vi "Test in Loop.vi"() -> ()   [LabVIEW 2025]
uses:
  99_Reference/LVMQTT-master/Controls/Connection_Return_Codes.ctl
  99_Reference/LVMQTT-master/Controls/User_Info.ctl
  99_Reference/LVMQTT-master/Controls/Connect_Flags.ctl
  99_Reference/LVMQTT-master/Controls/QoS.ctl
  99_Reference/LVMQTT-master/Controls/DUP_Flag.ctl
  99_Reference/LVMQTT-master/Controls/Retain_Flag.ctl
  <vilib>/NI/AMC/Read Termination Message.vi
  <vilib>/NI/AMC/Create Single Message.vi
  <vilib>/NI/AMC/Update Message Routing Info.vi
  <vilib>/NI/AMC/Globals.vi
  <vilib>/NI/AMC/Send Message.vi
  <vilib>/ErrorRing/Error Ring.xnode
  99_Reference/LVMQTT-master/MQTT_Functions.lvlib
  <vilib>/NI/AMC/AMC.lvlib
  <userlib>/_OpenG.lib/time/time.llb/openg_time.lvlib
panel:
  out "ReadCMD_0":string="\u0000\u0001{\"ID\": \"fc6981fe-2619-4699-a965-530b28fed39b\", \"TO\": \"0050C500001E\", \"FROM\": \"C87F542F1180\", \"CMD\": 0, \"CONTENT\": [{\"HOSTNAME\": \"SI-AGT01\", \"MAC\": \"0050C500001E\", \"IP\": \"172.16.0.248\", \"CENTER_NAME\": \"C87F542F1180\", \"ADD_TOPIC\": \"topic/PC/0050C500001E\", \"REQ_ID\": \"88519866-1952-4B11-8249-306205650CEC\"}], \"STATUS\": true, \"ERRCODE\": \"\", \"ERRMSG\": \"\", \"TIMESTAMP\": 175887754"
  in  "CMD_0":bool
  in  "Test Connect":bool
  out "Connection Status":T1
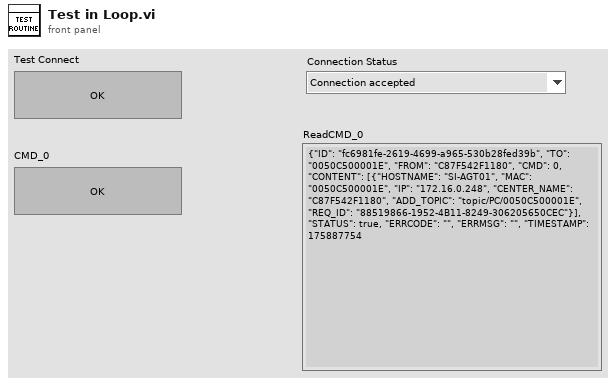
[diagram p1: front panel]
types:
  T1 = typedef "MQTT_Functions.lvlib/Connection_Return_Codes.ctl" = enum16{"Connection accepted", "Connection refused: unacceptable protocol version", "Connection refused: identifier rejected", "Connection refused: Server unavailable", "Connection refused: bad user name or password", "Connection refused: not authorized"}
  T2 = typedef "AMC.lvlib/Message Queue.ctl" = refnum<queue>
  T3 = typedef "MQTT_Functions.lvlib/QoS.ctl" = enum8{"At most once", "At least once", "Exactly once", "Reserved"}
  T4 = typedef "MQTT_Functions.lvlib/Retain_Flag.ctl" = bool
  T5 = typedef "MQTT_Functions.lvlib/DUP_Flag.ctl" = bool
  T6 = cluster{"Hostname":string, "Mac(From)":string, "IP":string, "ConnID":refnum<k5>}
  T7 = cluster{"QoS":T3, "DUP":T5, "Retain":T4, "Keep Alive (sec)":u16}
  T8 = typedef "MQTT_Functions.lvlib/Connect_Flags.ctl" = cluster{"user name":bool, "password":bool, "will retain":bool, "will flag":bool, "clean session":bool, "reserved":bool, "will QoS":T3}
  T9 = typedef "MQTT_Functions.lvlib/User_Info.ctl" = cluster{"User Name":string, "Password":string}
  T10 = cluster{"User Info":T9, "Client ID":string, "MQTT Broker":cluster{"address (IP)":string, "port":u16}, "Connection Status":T1, "Connect Flags":T8, "Connect Meta":cluster{"QoS":T3, "DUP":T5, "Retain":T4, "Keep Alive (sec)":u16}, "MainInfo":cluster{"Hostname":string, "Mac(From)":string, "IP":string, "ConnID":refnum<k5>}, "Topic":string, "tickCount":u32, "tickTarget":u32, "Message ID":u16}
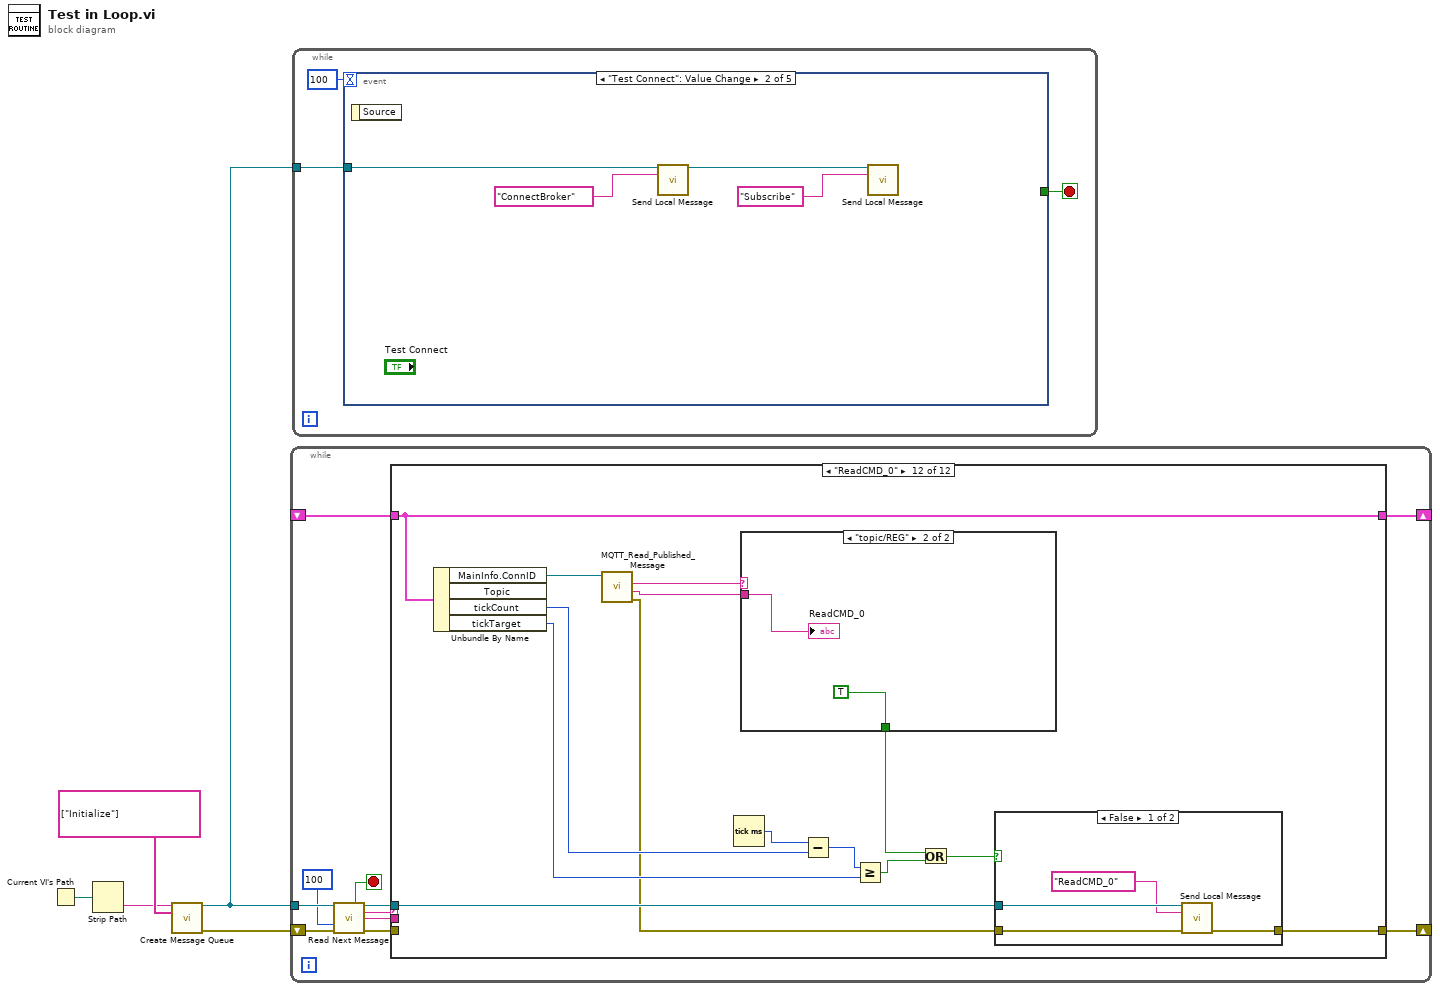
[diagram p0: block diagram]
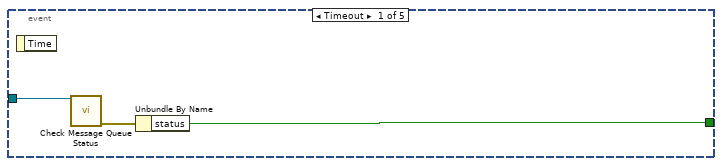
[diagram p2: hidden frame]
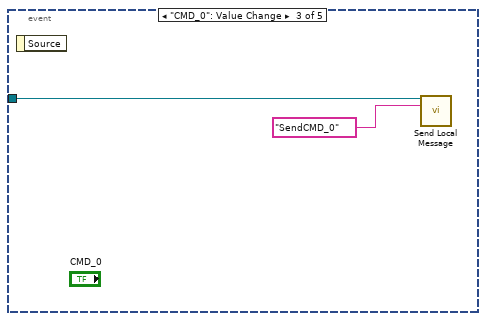
[diagram p3: hidden frame]
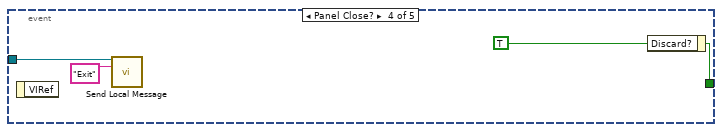
[diagram p4: hidden frame]
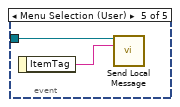
[diagram p5: hidden frame]
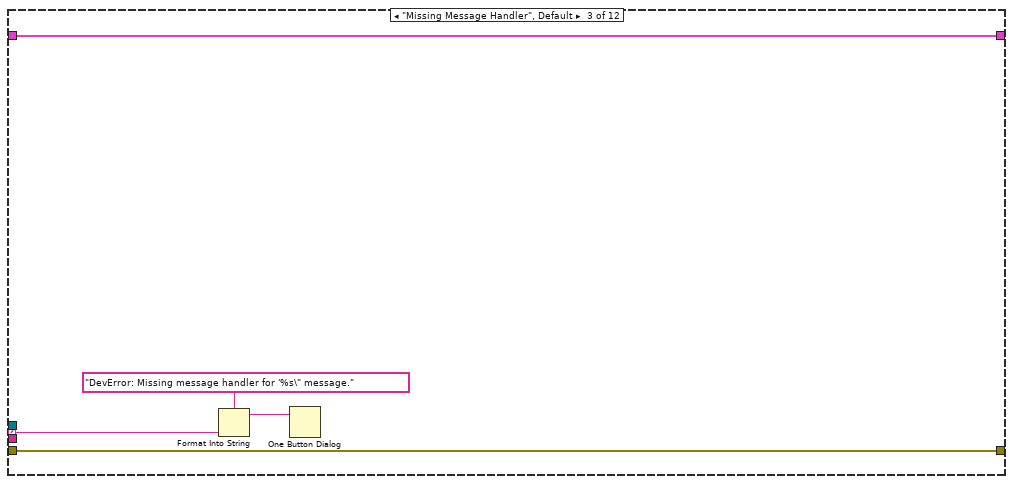
[diagram p8: hidden frame]
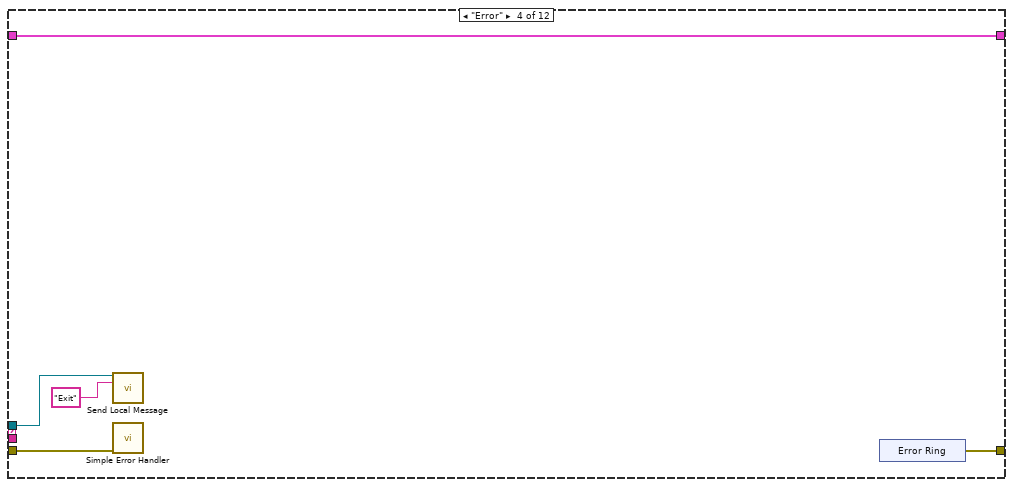
[diagram p9: hidden frame]
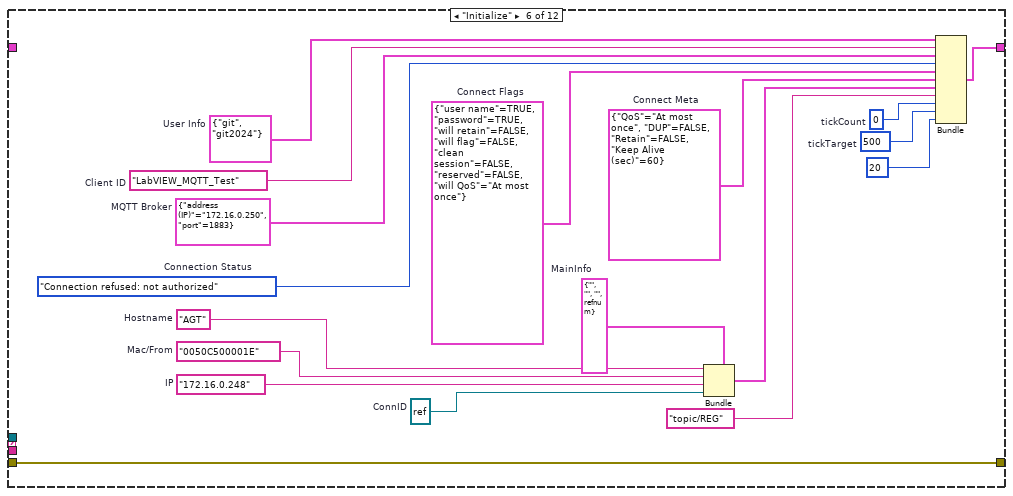
[diagram p11: hidden frame]
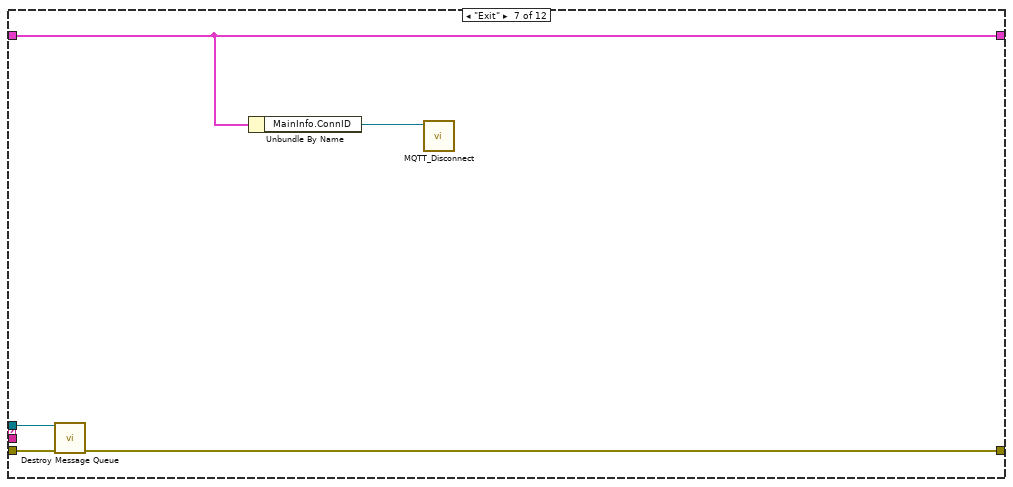
[diagram p12: hidden frame]
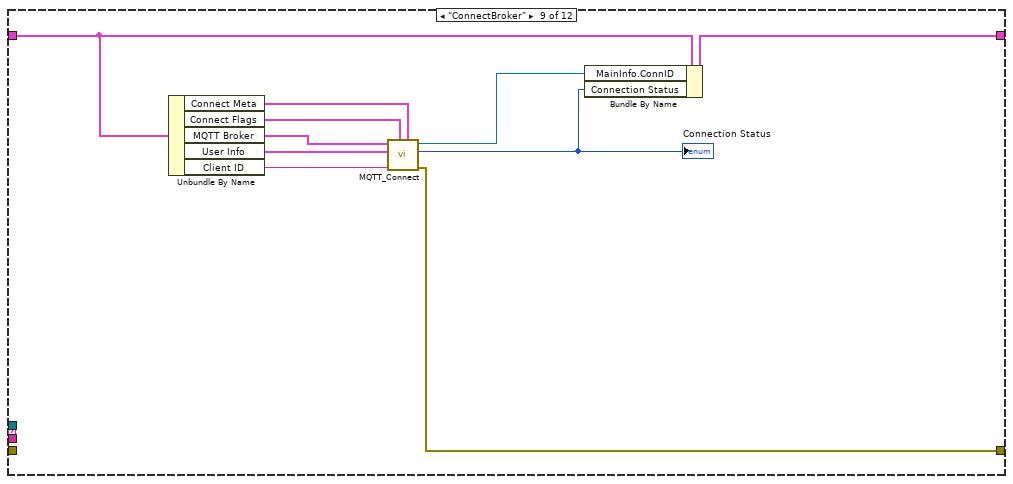
[diagram p14: hidden frame]
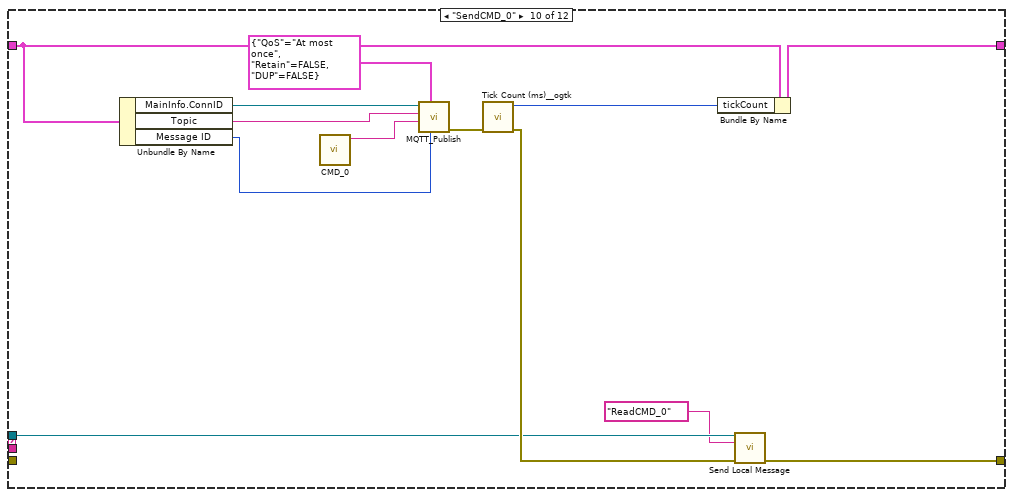
[diagram p15: hidden frame]
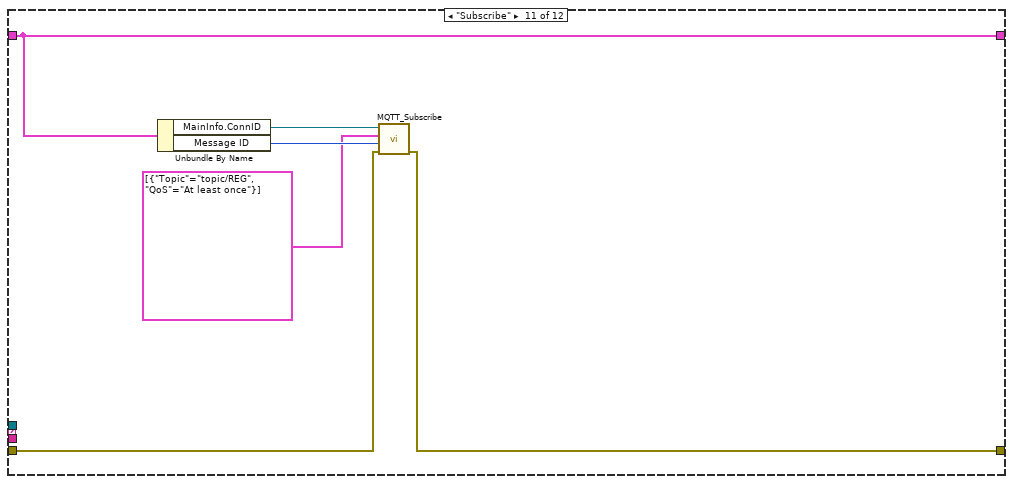
[diagram p16: hidden frame]
diagram:
  n1 = Current VI's Path() -> (path=w1:path)
  n2 = Strip Path(path=w1) -> (name=w4:string)  [unwired: 1 out]
  n3 = call <vilib>:"Create Message Queue.vi"("message queue name"=w4, "initial message names"=string[] ["Initialize"]) -> ("message queue out"=w3:T2, "error out"=w2:errorcluster)  [unwired: 12 in]
  n4 = while "Message Processor" {
    shift-left: w2 -> [w10]
    shift-right: [w14] -> _
    tunnel: w3 -> [w11]
    shift-left: _ -> [w16]
    shift-right: [w15] -> _
    stop <- w13 stop-if-true
    n5 = call <vilib>:"Read Next Message.vi"("message queue in"=w11, "timeout (1 ms)"=100 ("Timeout"), "error in"=w10) -> ("exit process?"=w13:bool, "message queue out"=w12:T2, "message name"=w8:string, "message value"=w7:string, "error out"=w9:errorcluster)  [unwired: 5 in, 3 out]
    n6 = case shown="\"ReadCMD_0\"" w8 {
      selector: w8 -> [_ _ w23 _ _ _ _ _ _ _ _ _]
      tunnel: [w18 w20 w25 w30 w33 w50 w53 w58 w63 w76 w87 w100] -> w15
      tunnel: w16 -> [w18 w20 w25 w30 w33 _ w53 w58 w68 w79 w87 w100]
      tunnel: w12 -> [_ _ _ w29 _ _ w55 _ _ w73 _ w98]
      tunnel: w9 -> [w17 w19 w24 w27 w32 w51 w56 w57 _ _ w85 _]
      tunnel: [w17 w19 w24 w26 w32 w51 w54 w57 w64 w70 w84 w99] -> w14
      tunnel: w7 -> [_ _ _ _ _ _ _ _ _ _ _ _]
      frame "---------- Framework Operations ----------" {
      }
      frame "", "Idle" {
      }
      frame "Missing Message Handler", Default {
        n7 = Format Into String(format string="DevError: Missing message handler for '%s\" message." ("message"), w23) -> (resulting string=w21:string)  [unwired: 2 in, 1 out]
        n8 = One Button Dialog(message=w21) -> ()  [unwired: 2 out]
      }
      frame "Error" {
        n9 = call <vilib>:"Send Local Message.vi"("message queue in"=w29, "message name"="Exit") -> ()  [unwired: 11 in, 3 out]
        n10 = call <vilib>:"Simple Error Handler.vi"("error in (no error)"=w27) -> ()  [unwired: 1 in, 8 out]
        n11 = xnode "Error Ring"() -> ("error out"=w26:errorcluster)
      }
      frame "---------- Generic Operations ----------" {
      }
      frame "Initialize" {
        w35 = u32 500  # tickTarget
        w36 = u32 0  # tickCount
        w38 = T6 {"Hostname"="", "Mac(From)"="", "IP"="", "ConnID"=refnum}  # MainInfo
        w39 = refnum<k5> refnum  # ConnID
        w42 = "0050C500001E"  # Mac/From
        w41 = "AGT"  # Hostname
        w43 = "172.16.0.248"  # IP
        w44 = T7 {"QoS"=enum."At most once", "DUP"=FALSE, "Retain"=FALSE, "Keep Alive (sec)"=60}  # Connect Meta
        w45 = T8 {"user name"=TRUE, "password"=TRUE, "will retain"=FALSE, "will flag"=FALSE, "clean session"=FALSE, "reserved"=FALSE, "will QoS"=enum."At most once"}  # Connect Flags
        w46 = Connection_Return_Codes."Connection refused: not authorized"  # Connection Status
        w47 = cluster{"address (IP)":string, "port":u16} {"address (IP)"="172.16.0.250", "port"=1883}  # MQTT Broker
        w48 = "LabVIEW_MQTT_Test"  # Client ID
        w49 = T9 {"User Name"="git", "Password"="git2024"}  # User Info
        n12 = Bundle(cluster=w38, "Hostname"=w41, "Mac(From)"=w42, "IP"=w43, "ConnID"=w39) -> (w40:T6)
        n13 = Bundle("User Info"=w49, "Client ID"=w48, "MQTT Broker"=w47, "Connection Status"=w46, "Connect Flags"=w45, "Connect Meta"=w44, "MainInfo"=w40, "Topic"="topic/REG", "tickCount"=w36, "tickTarget"=w35, "Message ID"=u16 20) -> (w50:T10)  [unwired: 1 in]
      }
      frame "Exit" {
        n14 = call <vilib>:"Destroy Message Queue.vi"("message queue in"=w55, "error in"=w56) -> ("error out"=w54:errorcluster)  [unwired: 11 in, 2 out]
        n15 = Unbundle By Name(w53) -> ("MainInfo.ConnID"=w52:refnum<k5>)
        n16 = call "MQTT_Disconnect.vi"("connection ID"=w52) -> ()  [unwired: 10 in, 1 out]
      }
      frame "---------- Application Operations ----------" {
        # "Dummy case to add a seperator in the Case Structure menu"
      }
      frame "ConnectBroker" {
        n17 = Unbundle By Name(w68) -> ("Connect Meta"=w61:T7, "Connect Flags"=w60:T8, "MQTT Broker"=w67:cluster{"address (IP)":string, "port":u16}, "User Info"=w66:T9, "Client ID"=w65:string)
        n18 = call "MQTT_Connect.vi"("Connect Meta"=w61, "Client ID"=w65, "Connect Flags"=w60, "User Info"=w66, "MQTT Broker"=w67) -> ("error out"=w64:errorcluster, "Connection Status"=w62:T1, "connection ID out"=w59:refnum<k5>)  [unwired: 4 in]
        "Connection Status" <- w62
        n19 = Bundle By Name(cluster=w68, "MainInfo.ConnID"=w59, "Connection Status"=w62) -> (w63:T10)
      }
      frame "SendCMD_0" {
        n20 = Unbundle By Name(w79) -> ("MainInfo.ConnID"=w81:refnum<k5>, "Topic"=w78:string, "Message ID"=w69:u16)
        n21 = call "CMD_0.vi"() -> ("JSON String"=w80:string)  [unwired: 11 in]
        n22 = call "MQTT_Publish.vi"("Message ID"=w69, "Publish Meta"=cluster{"QoS":T3, "Retain":T4, "DUP":T5} {"QoS"=enum."At most once", "Retain"=FALSE, "DUP"=FALSE}, "Message to be published"=w80, "Topic"=w78, "connection ID"=w81) -> ("error out"=w77:errorcluster)  [unwired: 5 in, 1 out]
        n23 = call <userlib>:"Tick Count (ms)__ogtk.vi"("error in (no error)"=w77) -> ("error out"=w74:errorcluster, "millisecond timer value"=w75:u32)  [unwired: 9 in]
        n24 = Bundle By Name(cluster=w79, "tickCount"=w75) -> (w76:T10)
        n25 = call <vilib>:"Send Local Message.vi"("message queue in"=w73, "message name"="ReadCMD_0", "error in"=w74) -> ("error out"=w70:errorcluster)  [unwired: 10 in, 2 out]
      }
      frame "Subscribe" {
        n26 = Unbundle By Name(w87) -> ("MainInfo.ConnID"=w86:refnum<k5>, "Message ID"=w83:u16)
        n27 = call "MQTT_Subscribe.vi"("error in (no error)"=w85, "Message ID"=w83, "Subscription Info Array"=cluster{"Topic":string, "QoS":T3}[] [{"Topic"="topic/REG", "QoS"=enum."At least once"}], "connection ID"=w86) -> ("error out"=w84:errorcluster)  [unwired: 6 in, 1 out]
      }
      frame "ReadCMD_0" {
        n28 = Unbundle By Name(w100) -> ("MainInfo.ConnID"=w101:refnum<k5>, "tickCount"=w96:u32, "tickTarget"=w94:u32)  [unwired: 1 out]
        n29 = call "MQTT_Read_Published_Message.vi"("connection ID"=w101) -> ("error out"=w89:errorcluster, "Message"=w88:string, "Topic Name"=w92:string)  [unwired: 5 in, 3 out]
        n30 = Tick Count (ms)() -> (millisecond timer value=w97:u32)
        n31 = case shown="\"topic/REG\"" w92 {
          tunnel: [_ TRUE] -> w90
          tunnel: w88 -> [_ w102]
          frame "False", Default {
          }
          frame "topic/REG" {
            "ReadCMD_0" <- w102
          }
        }
        n32 = Subtract(x=w97, y=w96) -> (x-y=w95:u32)
        n33 = Greater Or Equal?(x=w95, y=w94) -> (x >= y?=w93:bool)
        n34 = Or(x=w90, y=w93) -> (x .or. y?=w91:bool)
        n35 = case shown="False" w91 {
          tunnel: [w107 w108] -> w99
          tunnel: w98 -> [w106 _]
          tunnel: w89 -> [w104 w108]
          frame False {
            n36 = call <vilib>:"Send Local Message.vi"("message queue in"=w106, "message name"="ReadCMD_0", "error in"=w104) -> ("error out"=w107:errorcluster)  [unwired: 10 in, 2 out]
          }
          frame True {
          }
        }
      }
    }
  }
  n37 = while "Message Generator - User Interface Event Handler" {
    tunnel: w3 -> [w109]
    stop <- w110 stop-if-true
    n38 = event shown="[1] \"Test Connect\": Value Change" {
      selector: _ -> [_ _ _ _ _]
      dyn-events: _ -> [_ _ _ _ _]
      timeout: 100 ("Event Structure Timeout (ms)") -> [_ _ _ _ _]
      tunnel: [w112 _ _ w123 _] -> w110
      tunnel: w109 -> [w113 w118 w120 w121 w124]
      event Timeout {
        n39 = event-data() -> ()  [unwired: 2 out]
        n40 = call <vilib>:"Check Message Queue Status.vi"("message queue in"=w113) -> ("error out"=w114:errorcluster)  [unwired: 10 in, 4 out]
        n41 = Unbundle By Name(w114) -> ("status"=w112:bool)
      }
      event "Test Connect": Value Change {
        n42 = event-data() -> ()  [unwired: 2 out]
        n43 = call <vilib>:"Send Local Message.vi"("message queue in"=w118, "message name"="ConnectBroker") -> ("message queue out"=w115:T2)  [unwired: 11 in, 2 out]
        n44 = call <vilib>:"Send Local Message.vi"("message queue in"=w115, "message name"="Subscribe") -> ()  [unwired: 11 in, 3 out]
      }
      event "CMD_0": Value Change {
        n45 = event-data() -> ()  [unwired: 2 out]
        n46 = call <vilib>:"Send Local Message.vi"("message queue in"=w120, "message name"="SendCMD_0") -> ()  [unwired: 11 in, 3 out]
      }
      event Panel Close? {
        w123 = TRUE ("Discard?")
        n47 = event-data() -> ()  [unwired: 2 out]
        n48 = call <vilib>:"Send Local Message.vi"("message queue in"=w121, "message name"="Exit") -> ()  [unwired: 11 in, 3 out]
        n49 = event-data("Discard?"=w123) -> ()  [unwired: 1 in, 1 out]
      }
      event Menu Selection (User) {
        n50 = event-data() -> ("ItemTag"=w125:string)  [unwired: 1 out]
        n51 = call <vilib>:"Send Local Message.vi"("message queue in"=w124, "message name"=w125) -> ()  [unwired: 11 in, 3 out]
      }
    }
  }
